vi "Progetto SAM 2 - Andrea Alecce.vi"() -> ()   [LabVIEW 2018]
uses:
  <vilib>/sound2/lvsound2.llb/Sound Data Format.ctl
  <vilib>/sound2/lvsound2.llb/Sound Input Read (DBL).vi
  <vilib>/measure/maspectr.llb/FFT Spectrum (Mag-Phase) for N Chan.vi
  <vilib>/measure/NI_MAPro.lvlib
panel:
  out "File salvato in":path
  in  "Nome file":string="audio.log"
  out "Timestamp Pausa":timestamp
  in  "Stop":bool
  in  "Pause Button":bool
  in  "REC Button":bool
  in  "Canale Sorgente":u32
  in  "Formato Audio":T1={"sample rate (S/s)"=22050.0, "number of channels"=2, "bits per sample"=16}
  in  "Durata acquisizione (s)":dbl=1.0 min=0.1 step=0.1
  in  "Shuntdown Time":i32=-1 min=-1 step=1000
  in  "Soglia":dbl=0.0009999999999999996 step=0.0001
  out "Finestra di Errore":errorcluster
  out "Spettro":cluster{"f0":dbl, "df":dbl, "magnitude":dbl[]}[](graph)
  out "t0":timestamp[](array[timestamp])
  out "Signal":waveform(dbl)[](graph) caption="Waveform Graph"
  in  "Opzioni IIR":T2={"Topology"=enum."Butterworth", "Type"=enum."Lowpass", "Order"=1, "Lower Fc"=100.0, "Upper Fc"=200.0, "PB Ripple"=1.0, "SB Attenuation"=60.0} {"PB Ripple" format="%0.2f"; "SB Attenuation" format="%0.2f"; "Lower Fc" format="%0.2p"; "Upper Fc" format="%0.2p"}
  in  "optional IIR filter specifications":T3={"Lower PB"=100.0, "Upper PB"=0.0, "Lower SB"=200.0, "Upper SB"=0.0, "PB Gain"=-3.0, "SB Gain"=-60.0, "Scale"=TRUE} {"PB Gain" format="%0.2f"; "SB Gain" format="%0.2f"; "Lower SB" format="%0.2p"; "Upper SB" format="%0.2f"; "Lower PB" format="%0.2p"; "Upper PB" format="%0.2f"}
  out "IIR ON":bool
  out "FIR ON":bool
  in  "?":bool
  in  "optional FIR specifications":T4={"PB Gain"=-3.0, "SB Gain"=-60.0, "Scale"=TRUE, "Window"=enum."Flat Top"} {"SB Gain" format="%.2p"; "PB Gain" format="%.2p"}
  in  "Opzioni FIR":T5={"Topology"=enum."Off", "Type"=enum."Lowpass", "#Taps"=50, "Lower PB"=100.0, "Upper PB"=0.0, "Lower SB"=200.0, "Upper SB"=0.0} {"Lower SB" format="%0.2p"; "Upper SB" format="%0.2p"; "Lower PB" format="%0.2p"; "Upper PB" format="%0.2p"}
  out "n° chunck":i32
  out "Freq ad ampiezza max":string
  out "Ampiezza min":string
  out "Freq ad ampiezza min":string
  out "Ampiezza max":string
  out "Evento Audio":bool
  # "Filtraggio"
  # "Informazioni audio"
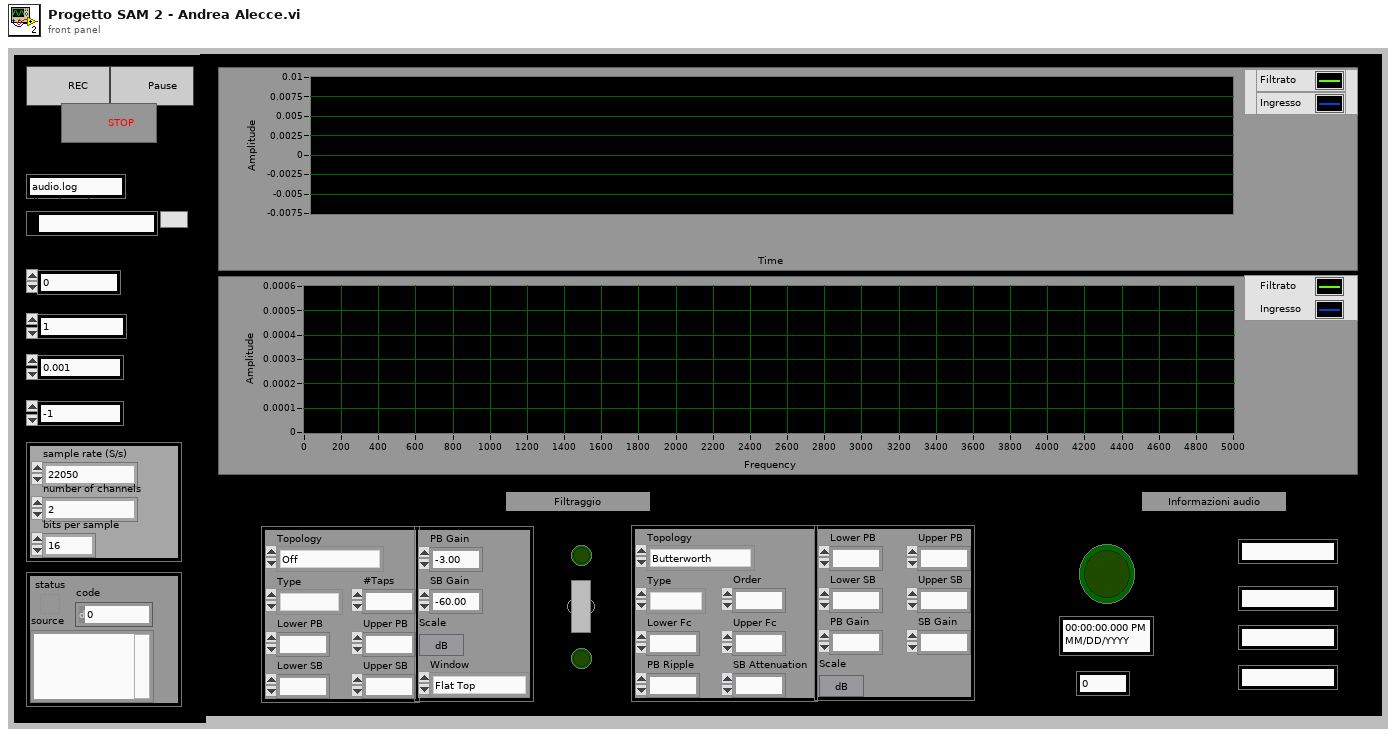
[diagram p1: front panel]
types:
  T1 = typedef "Sound Data Format.ctl" = cluster{"sample rate (S/s)":dbl, "number of channels":i32, "bits per sample":i32}
  T2 = cluster{"Topology":enum16{"Off", "Butterworth", "Chebyshev", "Inverse Chebyshev", "Elliptic", "Bessel"}, "Type":enum16{"Lowpass", "Highpass", "Bandpass", "Bandstop"}, "Order":i32, "Lower Fc":dbl, "Upper Fc":dbl, "PB Ripple":dbl, "SB Attenuation":dbl}
  T3 = cluster{"Lower PB":dbl, "Upper PB":dbl, "Lower SB":dbl, "Upper SB":dbl, "PB Gain":dbl, "SB Gain":dbl, "Scale":bool}
  T4 = cluster{"PB Gain":dbl, "SB Gain":dbl, "Scale":bool, "Window":enum16{"None", "Hanning", "Hamming", "Triangular", "Blackman", "Exact Blackman", "Blackman-Harris", "Kaiser-Bessel", "Flat Top"}}
  T5 = cluster{"Topology":enum16{"Off", "FIR by Specification", "Equi-ripple FIR", "Windowed FIR"}, "Type":enum16{"Lowpass", "Highpass", "Bandpass", "Bandstop"}, "#Taps":i32, "Lower PB":dbl, "Upper PB":dbl, "Lower SB":dbl, "Upper SB":dbl}
  T6 = cluster{"t0[0]":timestamp, "t0[1]":timestamp, "t0[2]":timestamp, "t0[3]":timestamp, "t0[4]":timestamp, "t0[5]":timestamp, "t0[6]":timestamp, "t0[7]":timestamp, "t0[8]":timestamp}
  T7 = typedef "Sound Input Task ID.ctl" = u32
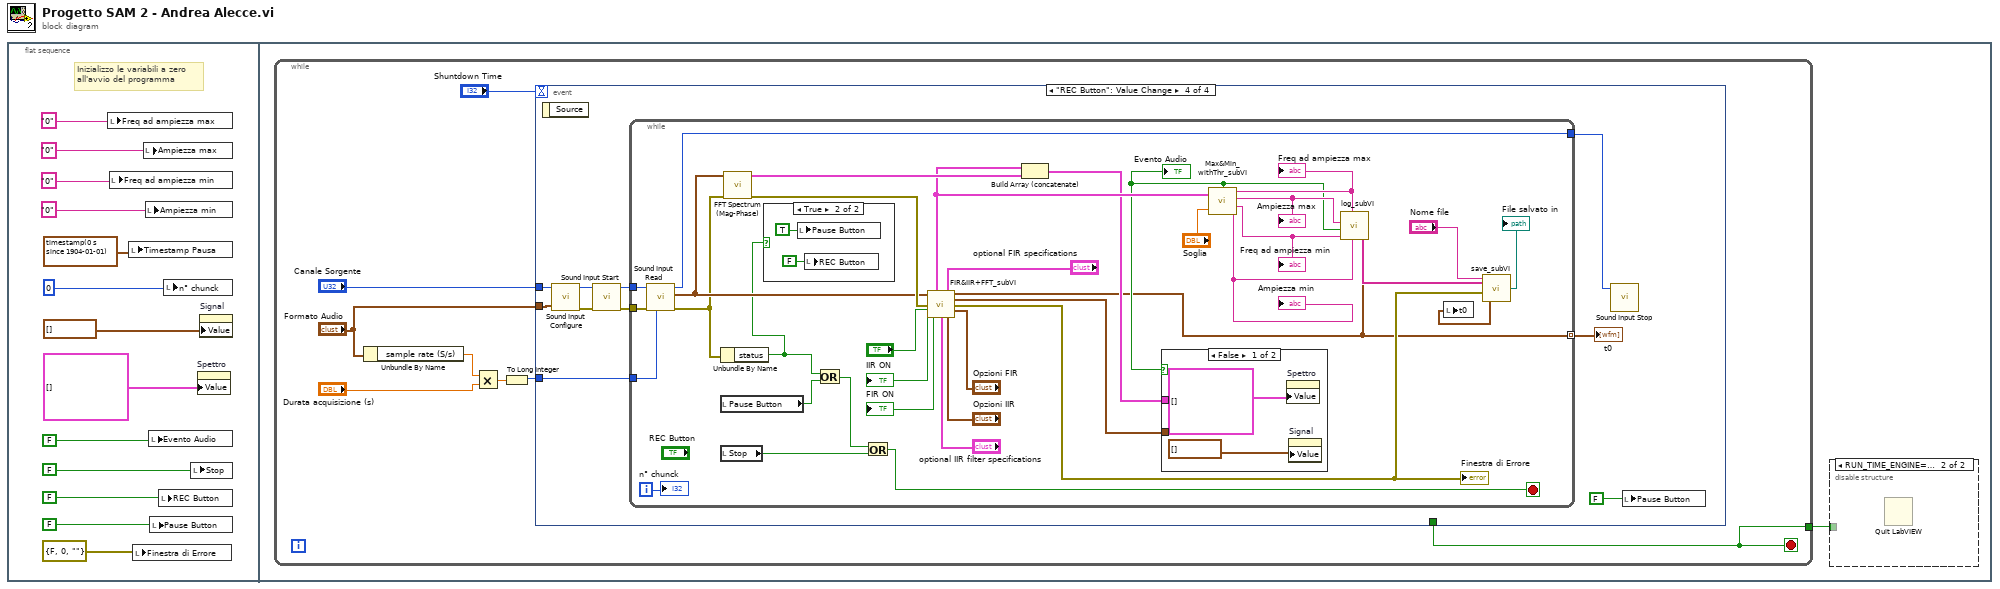
[diagram p0: block diagram]
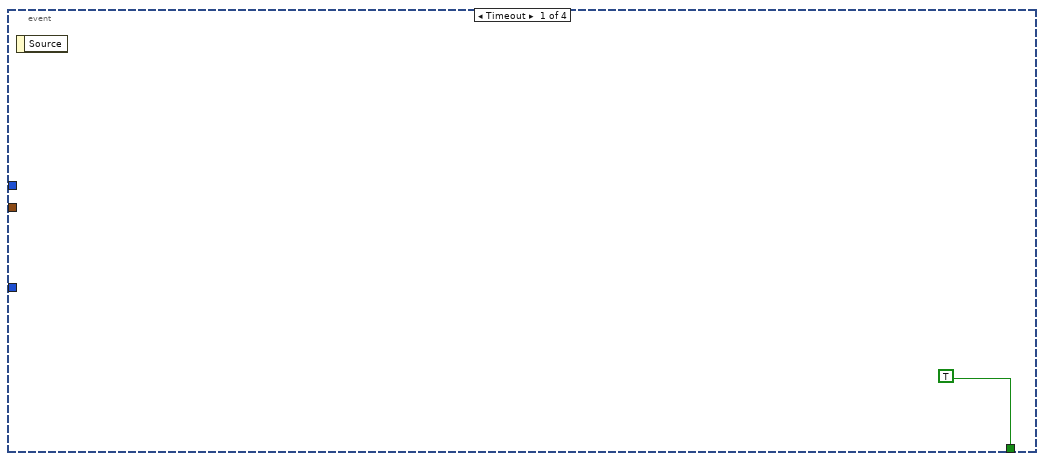
[diagram p3: hidden frame]
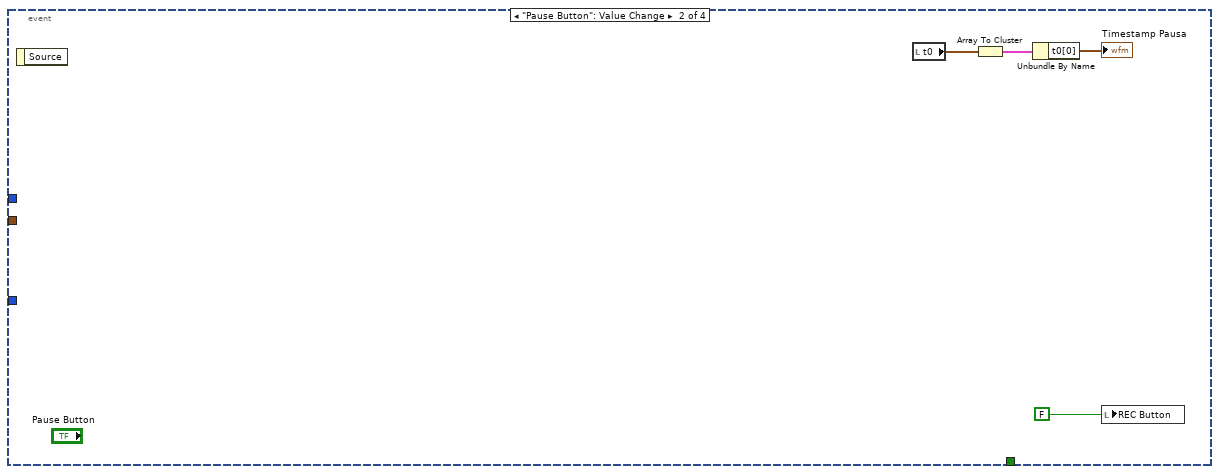
[diagram p4: hidden frame]
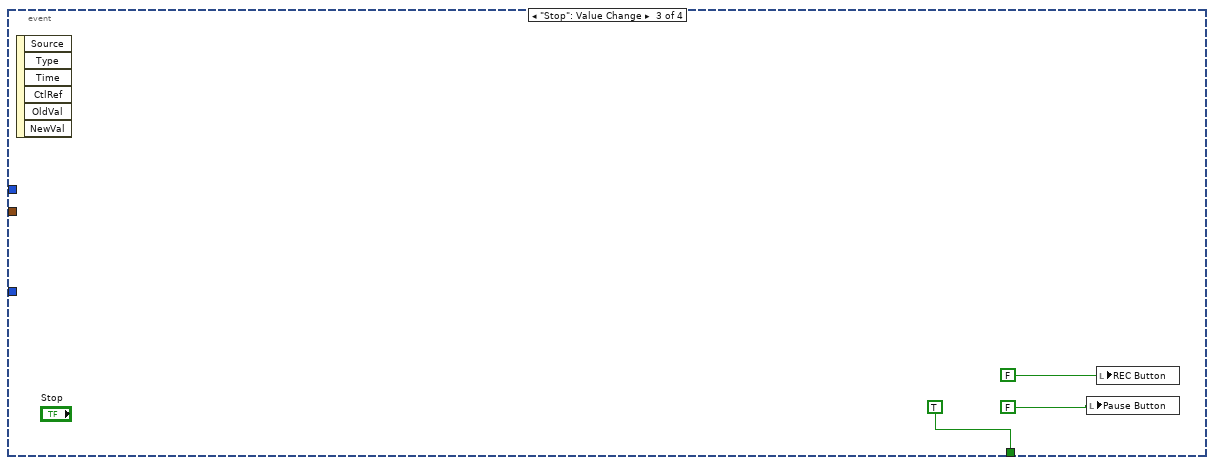
[diagram p5: hidden frame]
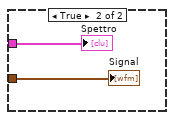
[diagram p7: hidden frame]
diagram:
  n1 = flat-sequence {
    frame #0 {
      # "Inizializzo le variabili a zero\nall'avvio del programma"
      n2 = local write "Freq ad ampiezza max"("0" ("Freq ad ampiezza max")) -> ()
      n3 = local write "Freq ad ampiezza min"("0" ("Freq ad ampiezza min")) -> ()
      n4 = local write "Timestamp Pausa"(timestamp(0 s since 1904-01-01)) -> ()
      n5 = local write "Finestra di Errore"(errorcluster {"status"=FALSE, "code"=0, "source"=""} ("Finestra di Errore")) -> ()
      n6 = local write "Ampiezza max"("0" ("Ampiezza max")) -> ()
      n7 = local write "Ampiezza min"("0" ("Ampiezza min")) -> ()
      n8 = local write "Evento Audio"(FALSE ("Evento Audio")) -> ()
      n9 = local write "Pause Button"(FALSE ("Pause Button")) -> ()
      n10 = local write "REC Button"(FALSE ("REC Button")) -> ()
      n11 = local write "n° chunck"(0 ("n° chunck")) -> ()
      n12 = local write "Stop"(FALSE ("Stop")) -> ()
      n13 = property on="Spettro" class="WFGraph (strict)"("Value"=cluster{"f0":dbl, "df":dbl, "magnitude":dbl[]}[] [] ("Spettro")) -> ()  [unwired: 2 in, 2 out]
      n14 = property on="Signal" class="WFGraph (strict)"("Value"=waveform(dbl)[] [] ("Signal")) -> ()  [unwired: 2 in, 2 out]
    }
    frame #1 {
      n15 = while {
        tunnel: [w18] -> w14
        stop <- w18 stop-if-true
        n16 = Unbundle By Name("Formato Audio") -> ("sample rate (S/s)"=w22:dbl)
        n17 = Multiply(x=w22, y="Durata acquisizione (s)") -> (x*y=w20:dbl)
        n18 = To Long Integer(number=w20) -> (32bit integer=w19:i32)
        n19 = event shown="[3] \"REC Button\": Value Change" {
          selector: _ -> [_ _ _ _]
          dyn-events: _ -> [_ _ _ _]
          timeout: "Shuntdown Time" -> [_ _ _ _]
          tunnel: [TRUE _ TRUE _] -> w18
          tunnel: w19 -> [_ _ _ w40]
          tunnel: "Formato Audio" -> [_ _ _ w35]
          tunnel: "Canale Sorgente" -> [_ _ _ w34]
          event Timeout {
            n20 = event-data() -> ()  [unwired: 1 in, 1 out]
          }
          event "Pause Button": Value Change {
            n21 = event-data() -> ()  [unwired: 1 in, 1 out]
            n22 = local read "t0"() -> (w26:timestamp[])
            n23 = Array To Cluster(array=w26) -> (cluster=w25:T6)
            n24 = Unbundle By Name(w25) -> ("t0[0]"=→"Timestamp Pausa":timestamp)
            n25 = local write "REC Button"(FALSE ("Record Button")) -> ()
          }
          event "Stop": Value Change {
            n26 = event-data() -> ()  [unwired: 1 in, 6 out]
            n27 = local write "Pause Button"(FALSE ("Stop REC")) -> ()
            n28 = local write "REC Button"(FALSE ("Record Button")) -> ()
          }
          event "REC Button": Value Change {
            n29 = event-data() -> ()  [unwired: 1 in, 1 out]
            n30 = call <vilib>:"Sound Input Configure.vi"("sound format"=w35, "device ID"=w34) -> ("error out"=w32:errorcluster, "task ID"=w33:T7)  [unwired: 8 in]
            n31 = call <vilib>:"Sound Input Start.vi"("error in (no error)"=w32, "task ID"=w33) -> ("error out"=w37:errorcluster, "task ID out"=w36:T7)  [unwired: 8 in]
            n32 = while {
              tunnel: [w76] -> w39
              tunnel: [w41] -> w31 mode=indexing
              tunnel: w40 -> [w75]
              tunnel: w37 -> [w74]
              tunnel: w36 -> [w73]
              i -> [w72]
              stop <- w71 stop-if-true
              n33 = call-poly <vilib>:"Sound Input Read.vi"("number of samples/ch"=w75, "error in (no error)"=w74, "task ID"=w73) -> ("error out"=w48:errorcluster, "data"=w53:waveform(dbl)[], "task ID out"=w76:T7)  [unwired: 6 in]
              n34 = Unbundle By Name(w48) -> ("status"=w47:bool)
              n35 = local read "Pause Button"() -> (w55:bool)
              n36 = local read "Stop"() -> (w54:bool)
              n37 = call-poly <vilib>:"FFT Spectrum (Mag-Phase).vi"("error in (no error)"=w48, "time signals"=w53) -> ("error out"=w62:errorcluster, "magnitudes"=w63:cluster{"f0":dbl, "df":dbl, "magnitude":dbl[]}[])  [unwired: 5 in, 3 out]
              n38 = case shown="True" w47 {
                frame False {
                }
                frame True {
                  n39 = local write "Pause Button"(TRUE ("Pause Button")) -> ()
                  n40 = local write "REC Button"(FALSE ("REC Button")) -> ()
                }
              }
              n41 = Or(x=w47, y=w55) -> (x .or. y?=w70:bool)
              n42 = Or(x=w70, y=w54) -> (x .or. y?=w71:bool)
              n43 = call "FIR&IIR+FFT_subVI.vi"("waveform array IN"=w53, "optional FIR filter specifications"="optional FIR specifications", "error in (no error)"=w62, "FIR / IIR"="?", "FIR filter specifications"="Opzioni FIR", "optional IIR filter specifications"="optional IIR filter specifications", "IIR filter specifications"="Opzioni IIR") -> ("magnitude"=w61:cluster{"f0":dbl, "df":dbl, "magnitude":dbl[]}, "t0"=w41:timestamp, "FIR ON"=→"FIR ON":bool, "Signal"=w50:waveform(dbl)[], "error out"=w43:errorcluster, "IIR ON"=→"IIR ON":bool)  [unwired: 3 in]
              "Finestra di Errore" <- w43
              n44 = Build Array (concatenate)(w61, w63) -> (w49:cluster{"f0":dbl, "df":dbl, "magnitude":dbl[]}[])
              n45 = call "Max&Min_withThr_subVI.vi"("Soglia"="Soglia", "magnitude"=w61) -> ("Ampiezza min"=w59:string, "freq ad ampiezza min"=w58:string, "Ampiezza max"=w56:string, "freq ad ampiezza max"=w57:string, "OverThr"=w51:bool)
              "Evento Audio" <- w51
              "Ampiezza min" <- w59
              "Ampiezza max" <- w56
              "Freq ad ampiezza min" <- w58
              "Freq ad ampiezza max" <- w57
              n46 = case shown="False" w51 {
                tunnel: w50 -> [_ w82]
                tunnel: w49 -> [_ w81]
                frame False {
                  n47 = property on="Spettro" class="WFGraph (strict)"("Value"=cluster{"f0":dbl, "df":dbl, "magnitude":dbl[]}[] [] ("Spettro")) -> ()  [unwired: 2 in, 2 out]
                  n48 = property on="Signal" class="WFGraph (strict)"("Value"=waveform(dbl)[] [] ("Signal")) -> ()  [unwired: 2 in, 2 out]
                }
                frame True {
                  "Signal" <- w82
                  "Spettro" <- w81
                }
              }
              n49 = call "log_subVI.vi"("time stamp"=w41, "Ampiezza Min"=w59, "freq ad ampiezza max"=w57, "freq ad ampiezza min"=w58, "Boolean 2"=w51, "Ampiezza Max"=w56) -> ("Formatted String Output"=w46:string[])  [unwired: 1 in]
              n50 = call "save_subVI.vi"("input cluster"=w43, "array"=w46, "Nome file"="Nome file") -> ("File salvato in"=→"File salvato in":path, "t0"=w44:timestamp[])
              n51 = local write "t0"(w44) -> ()
              "n° chunck" <- w72
            }
            "t0" <- w31
            n52 = call <vilib>:"Sound Input Stop.vi"("task ID"=w39) -> ()  [unwired: 9 in, 2 out]
            n53 = local write "Pause Button"(FALSE ("Stop REC")) -> ()
          }
        }
      }
      n54 = disable-structure shown="RUN_TIME_ENGINE==True" {
        disable-tunnel: w14 -> [_ _]
        frame condition #0 (active) {
        }
        frame condition #1 {
          n55 = Quit LabVIEW() -> ()  [unwired: 1 in]
        }
      }
    }
  }
